vi "Container To String.vi"(0 "variant":variant, 11 "error in (no error)":errorcluster) -> (4 "string":string, 6 "label":string, 15 "error out":errorcluster)   [LabVIEW 2015, in "LV String Utils v1.lvlib"]
doc: "Converts anything to string. String representation is as much compatible with Python repr as possible. Additionally returns label of the wire which is provided at the input."
uses:
  LV String Utils v1.lvlib
  <vilib>/Utility/error.llb/Error Cluster From Error Code.vi
  <vilib>/ErrorRing/Error Ring.xnode
  <vilib>/Utility/Data Type/NI_Data Type.lvlib
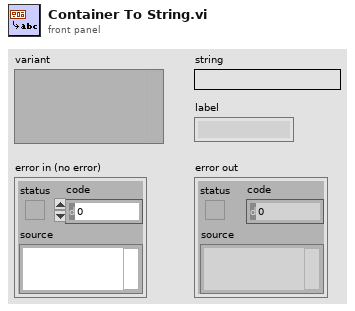
[diagram p1: front panel]
types:
  T1 = typedef "NI_Data Type.lvlib/Data Type.ctl" = enum8{"Invalid Type", "Void", "I8", "I16", "I32", "I64", "U8", "U16", "U32", "U64", "Single Float", "Double Float", "Extended Float", "Single Complex", "Double Complex", "Extended Complex", "Enum U8", "Enum U16", "Enum U32", "Enum U64", "Single Float With Unit", "Double Float With Unit", "Extended Float With Unit", "Single Complex with Unit", "Double Complex with Unit", "Extended Complex with Unit", "Boolean", "String", "Path", "Picture", "Tag", "Array", "Cluster", "Variant", "LV Variant", "Waveform", "Timestamp", "Digital Waveform", "Digital Data", "ExpressData", "Refnum", "External Data", "VI", "Poly VI", "LabVIEW Class Instance", "Fixed Point"}
  T2 = typedef "Refnum Subtype Enum__ogtk.ctl" = enum8{"Generic", "Datalog File Refnum", "Byte Stream File Refnum", "Device Refnum", "Occurence Refnum", "TCP Connection Refnum", "VISA Refnum (Obsolete)", "Automation Renum", "VI Server Refnum", "Menu Refnum", "IVI Refnum (Obsolete)", "IMAQ Session", "0x0C", "Datasocket Refnum", "VISA Resource", "IVI Logical Name", "UDP Connection Refnum", "Notifier Refnum", "Queue Refnum", "IrDA Refnum", "Hardware Plugin Refnum", "Hardware Plugin Tag Refnum", "DAQmx Refnum", "Event Registration Refnum", ".NET Refnum", "User Event Refnum", "0x1A", "Event Callback", "0x1C", "0x1D", "Only Used Internal to LabVIEW", "Bluetooth", "Data Value References", "RT FIFO", "TDM Streaming"}
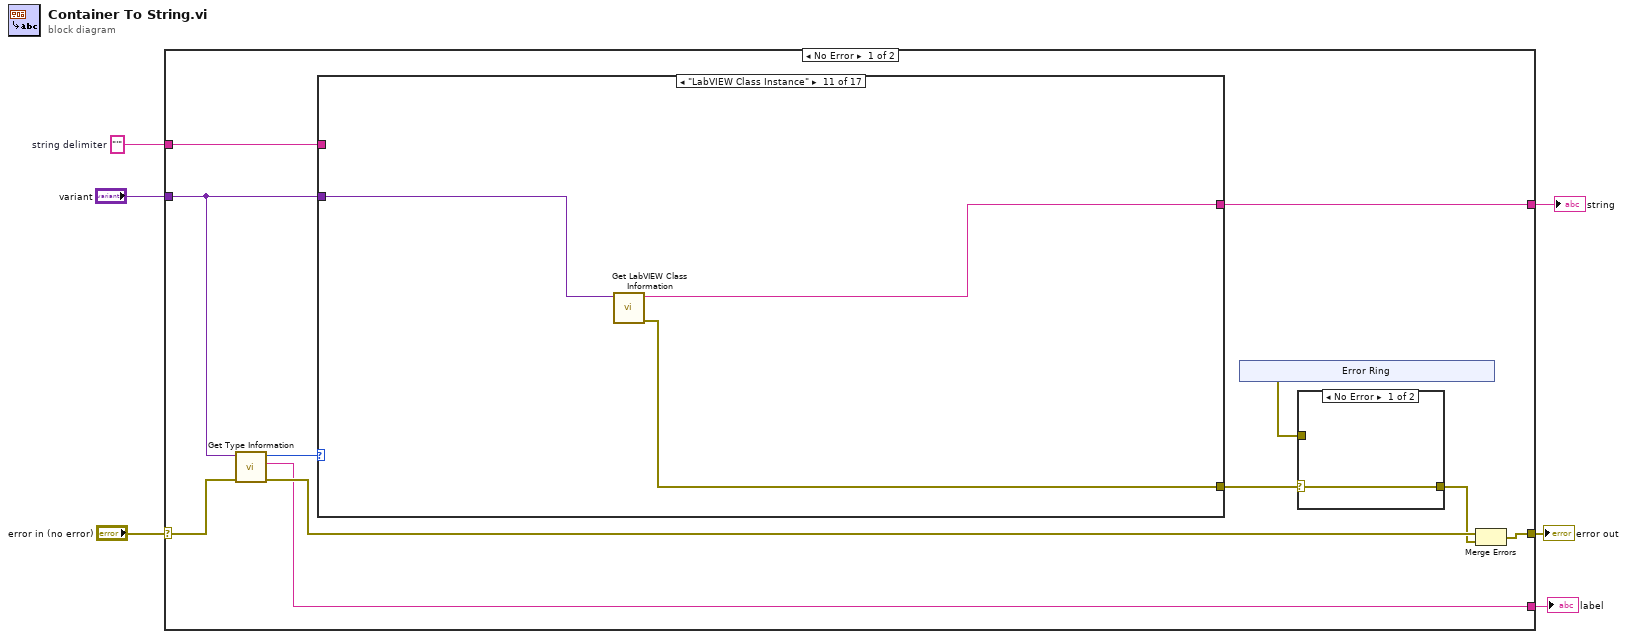
[diagram p0: block diagram]
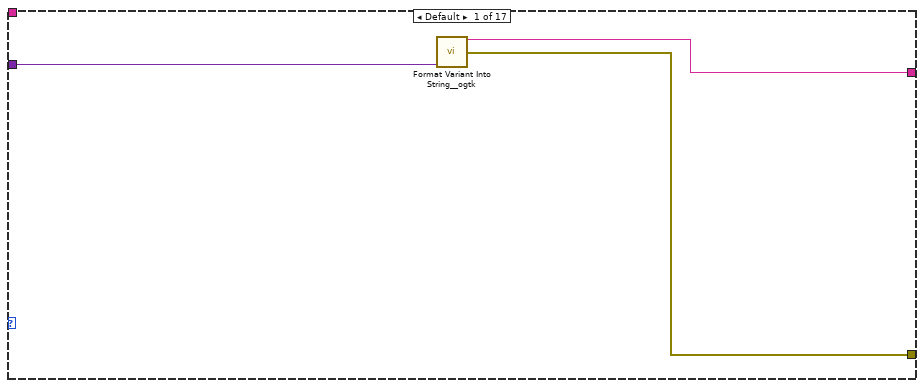
[diagram p3: hidden frame]
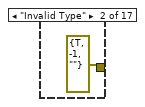
[diagram p4: hidden frame]
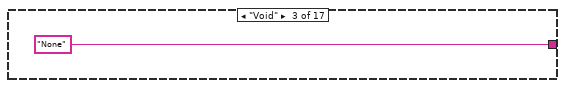
[diagram p5: hidden frame]
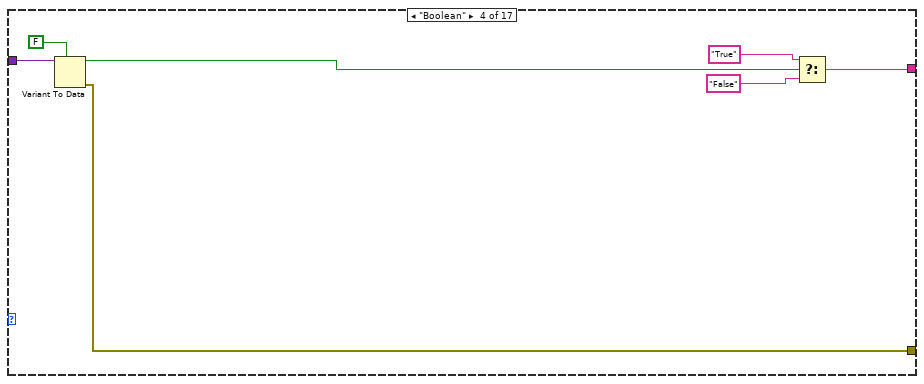
[diagram p6: hidden frame]
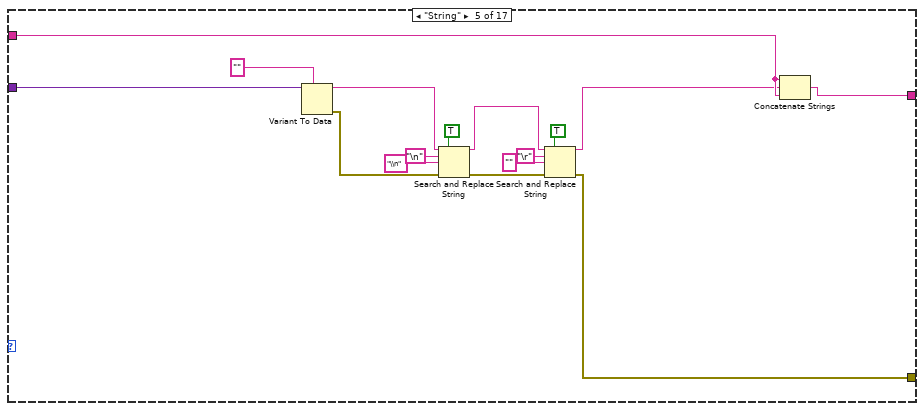
[diagram p7: hidden frame]
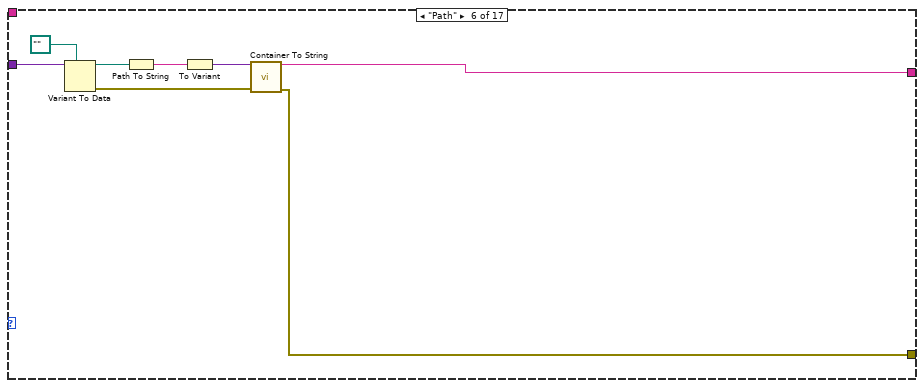
[diagram p8: hidden frame]
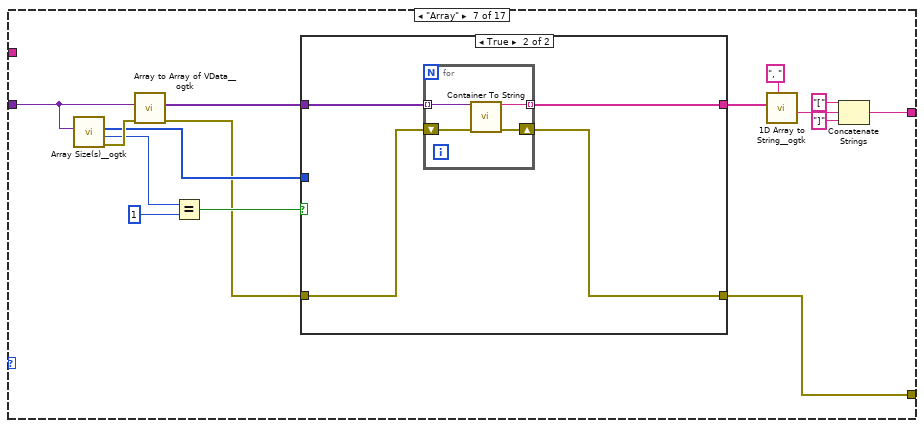
[diagram p9: hidden frame]
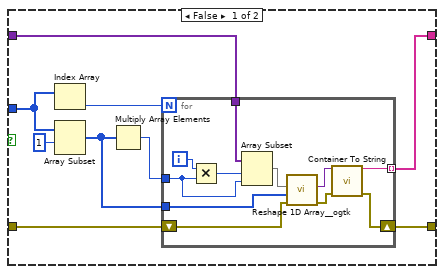
[diagram p10: hidden frame]
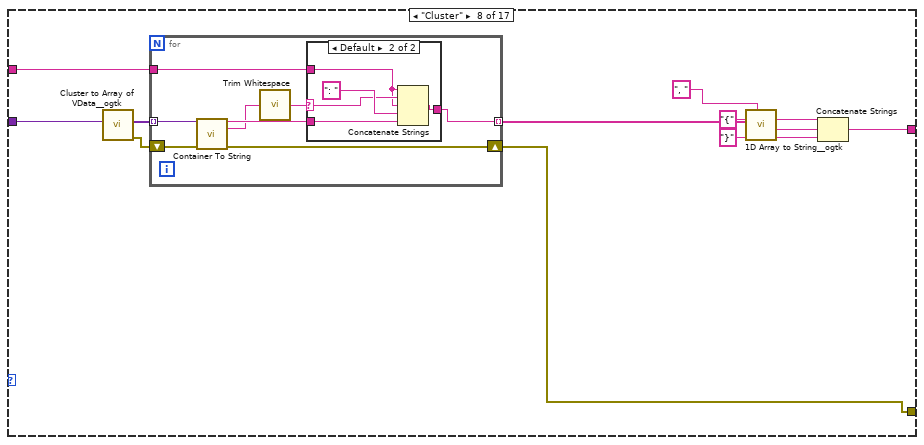
[diagram p11: hidden frame]
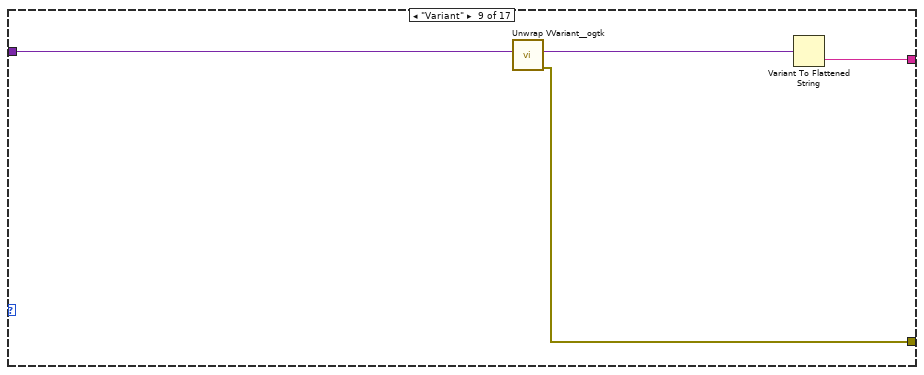
[diagram p13: hidden frame]
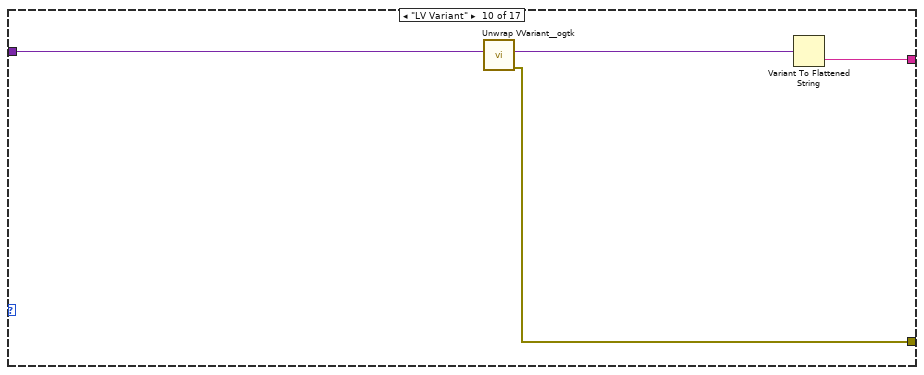
[diagram p14: hidden frame]
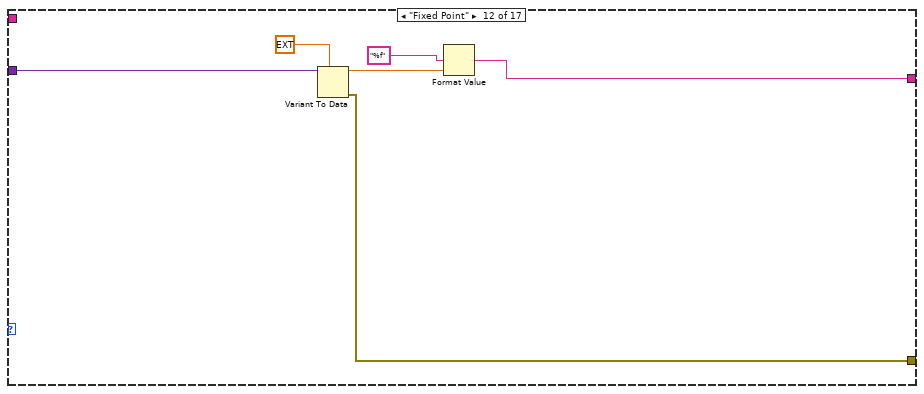
[diagram p15: hidden frame]
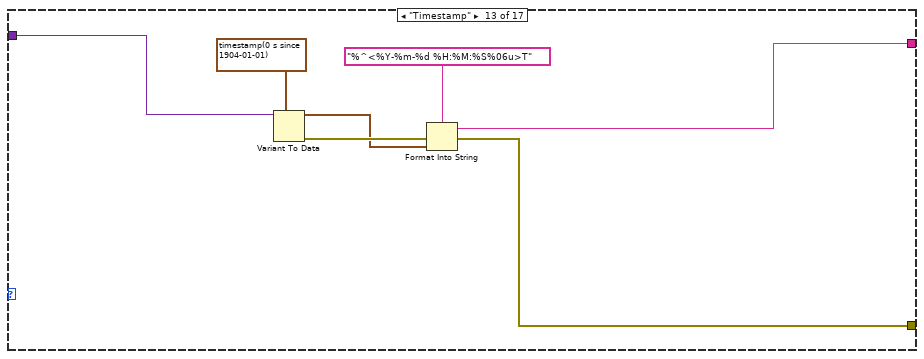
[diagram p16: hidden frame]
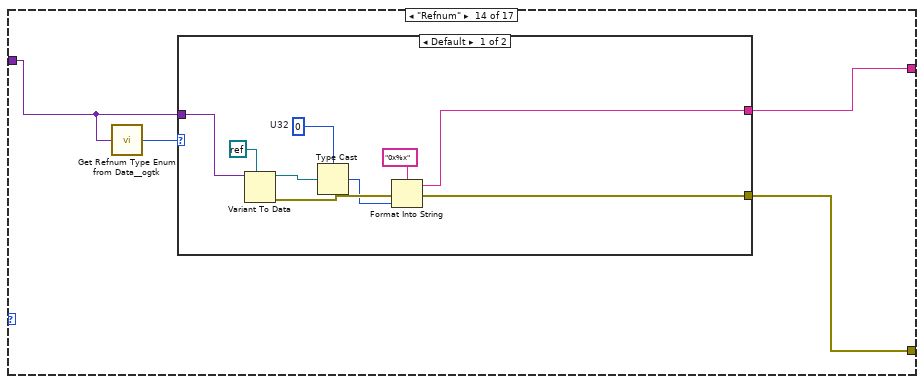
[diagram p17: hidden frame]
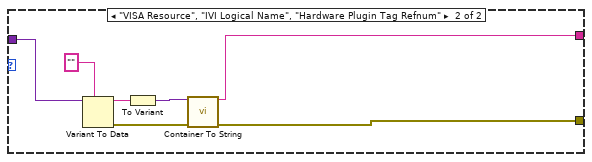
[diagram p18: hidden frame]
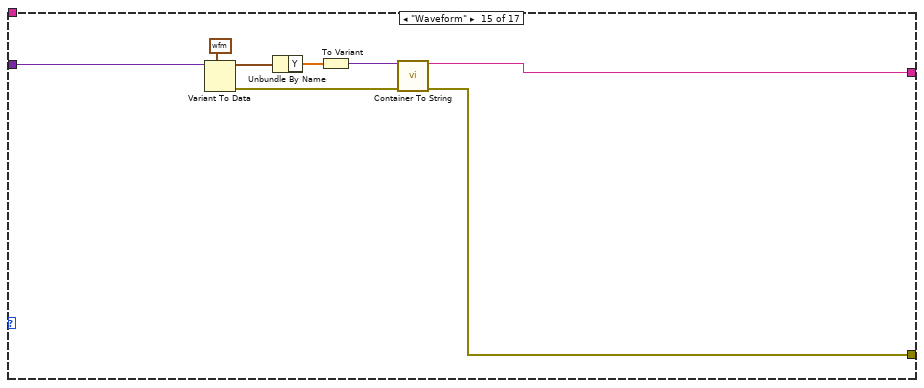
[diagram p19: hidden frame]
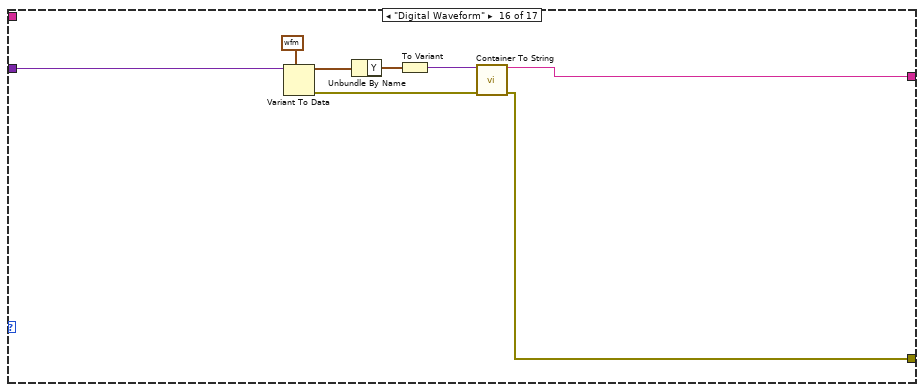
[diagram p20: hidden frame]
diagram:
  w2 = "'"  # string delimiter
  n1 = case shown="No Error" "error in (no error)" {
    selector: "error in (no error)" -> [w10 w196]
    tunnel: [w16 _] -> w6
    tunnel: "variant" -> [w15 _]
    tunnel: [w13 w196] -> w4
    tunnel: [w12 _] -> w3
    tunnel: w2 -> [w11 _]
    frame No Error {
      n2 = call <vilib>:"Get Type Information.vi"("error in (no error)"=w10, "Variant"=w15) -> ("error out"=w14:errorcluster, "Name"=w12:string, "Type"=w17:T1)  [unwired: 5 in, 2 out]
      n3 = case shown="\"LabVIEW Class Instance\"" w17 {
        tunnel: w15 -> [w26 _ _ w34 w51 w58 w66 w108 w130 w134 w137 w144 w150 w155 w179 w183 w194]
        tunnel: [w24 _ "None" ("output string") w32 w49 w54 w65 w104 w131 w135 w136 w140 w145 w153 w172 w180 w188] -> w16
        tunnel: [w25 errorcluster {"status"=TRUE, "code"=-1, "source"=""} ("error out") _ w29 w39 w52 w60 w105 w128 w132 w138 w139 w146 w152 w173 w181 w189] -> w9
        tunnel: w11 -> [_ _ _ _ w48 _ _ w103 _ _ _ _ _ _ _ _ _]
        frame Default {
          n4 = call <userlib>:"Format Variant Into String__ogtk.vi"("Variant"=w26) -> ("Output String"=w24:string, "error out"=w25:errorcluster)  [unwired: 13 in]
        }
        frame "Invalid Type" {
        }
        frame "Void" {
        }
        frame "Boolean" {
          n5 = Variant To Data(type=FALSE, Variant=w34) -> (data=w33:bool, error out=w29:errorcluster)  [unwired: 1 in]
          n6 = Select(t="True", s=w33, f="False") -> (s? t:f=w32:string)
        }
        frame "String" {
          n7 = Variant To Data(type="", Variant=w51) -> (data=w38:string, error out=w40:errorcluster)  [unwired: 1 in]
          n8 = Search and Replace String(replace all?=TRUE ("replace all? (F)"), input string=w38, search string="\n", replace string="\\n" ("replace string (\"\")"), error in=w40) -> (result string=w37:string, error out=w41:errorcluster)  [unwired: 3 in, 2 out]
          n9 = Search and Replace String(replace all?=TRUE ("replace all? (F)"), input string=w37, search string="\r", replace string="" ("replace string (\"\")"), error in=w41) -> (result string=w36:string, error out=w39:errorcluster)  [unwired: 3 in, 2 out]
          n10 = Concatenate Strings(w48, w36, w48) -> (w49:string)
        }
        frame "Path" {
          n11 = Variant To Data(type=path "", Variant=w58) -> (data=w57:path, error out=w53:errorcluster)  [unwired: 1 in]
          n12 = Path To String(path=w57) -> (string=w56:string)
          n13 = To Variant(anything=w56) -> (Variant=w55:variant)
          n14 = call "Container To String.vi"("variant"=w55, "error in (no error)"=w53) -> ("string"=w54:string, "error out"=w52:errorcluster)  [unwired: 11 in, 1 out]
        }
        frame "Array" {
          n15 = call <userlib>:"Array Size(s)__ogtk.vi"("Array"=w66) -> ("error out"=w68:errorcluster, "N dims"=w63:u32, "Size(s)"=w62:u32[])  [unwired: 8 in]
          n16 = call <userlib>:"Array to Array of VData__ogtk.vi"("error in (no error)"=w68, "MultiD Array"=w66) -> ("error out"=w61:errorcluster, "1D Array of Variants"=w69:variant[])  [unwired: 8 in]
          n17 = Equal?(x=w63, y=u32 1) -> (x = y?=w64:bool)
          n18 = case shown="True" w64 {
            tunnel: w69 -> [w83 w98]
            tunnel: w62 -> [w78 _]
            tunnel: [w82 w97] -> w74
            tunnel: w61 -> [w76 w96]
            tunnel: [w75 w95] -> w60
            frame False {
              n19 = Index Array(array=w78) -> (element=w79:u32)  [unwired: 1 in]
              n20 = Array Subset(array=w78, index=1) -> (w77:u32[])  [unwired: 1 in]
              n21 = Multiply Array Elements(1:w77) -> (0:w80:u32)
              n22 = for {
                N: w79 -> [_]
                tunnel: w83 -> [w94]
                tunnel: [w91] -> w82 mode=indexing
                tunnel: w77 -> [w89]
                tunnel: w80 -> [w87]
                shift-right: [w84] -> w75
                shift-left: w76 -> [w85]
                i -> [w93]
                n23 = Multiply(x=w93, y=w87) -> (x*y=w92:u32)
                n24 = Array Subset(array=w94, index=w92, length=w87) -> (w90:variant[])
                n25 = call <userlib>:"Reshape 1D Array__ogtk.vi"("error in (no error)"=w85, "Size(s)"=w89, "1D Array"=w90) -> ("error out"=w86:errorcluster, "Reshaped VArray"=w88:variant)  [unwired: 7 in]
                n26 = call "Container To String.vi"("variant"=w88, "error in (no error)"=w86) -> ("string"=w91:string, "error out"=w84:errorcluster)  [unwired: 11 in, 1 out]
              }
            }
            frame True {
              n27 = for {
                tunnel: w98 -> [w102] mode=indexing
                tunnel: [w101] -> w97 mode=indexing
                shift-right: [w100] -> w95
                shift-left: w96 -> [w99]
                n28 = call "Container To String.vi"("variant"=w102, "error in (no error)"=w99) -> ("string"=w101:string, "error out"=w100:errorcluster)  [unwired: 11 in, 1 out]
              }
            }
          }
          n29 = call <userlib>:"1D Array to String__ogtk.vi"("delimiter (Tab)"=", ", "Array of Strings"=w74) -> ("delimited string"=w72:string)  [unwired: 9 in]
          n30 = Concatenate Strings("[" ("string"), w72, "]" ("string")) -> (w65:string)
        }
        frame "Cluster" {
          n31 = call <userlib>:"Cluster to Array of VData__ogtk.vi"("Cluster"=w108) -> ("error out"=w106:errorcluster, "Array of VData"=w107:variant[])  [unwired: 9 in]
          n32 = for {
            tunnel: w107 -> [w121] mode=indexing
            tunnel: [w117] -> w113 mode=indexing
            shift-right: [w120] -> w105
            shift-left: w106 -> [w119]
            tunnel: w103 -> [w114]
            n33 = call "Container To String.vi"("variant"=w121, "error in (no error)"=w119) -> ("string"=w118:string, "label"=w115:string, "error out"=w120:errorcluster)  [unwired: 11 in]
            n34 = call <vilib>:"Trim Whitespace.vi"("string"=w115) -> ("trimmed string"=w116:string)  [unwired: 1 in]
            n35 = case shown="Default" w116 {
              selector: w116 -> [_ w124]
              tunnel: w118 -> [w122 w127]
              tunnel: [w122 w126] -> w117
              tunnel: w114 -> [_ w123]
              frame "" {
              }
              frame Default {
                n36 = Concatenate Strings(w123, w124, w123, ": " ("string"), w127) -> (w126:string)
              }
            }
          }
          n37 = call <userlib>:"1D Array to String__ogtk.vi"("delimiter (Tab)"=", ", "Array of Strings"=w113) -> ("delimited string"=w111:string)  [unwired: 9 in]
          n38 = Concatenate Strings("{" ("string"), w111, "}" ("string")) -> (w104:string)
        }
        frame "Variant" {
          n39 = call <userlib>:"Unwrap VVariant__ogtk.vi"("VVariant"=w130) -> ("error out"=w128:errorcluster, "Variant"=w129:variant)  [unwired: 9 in]
          n40 = Variant To Flattened String(Variant=w129) -> (data string=w131:string)  [unwired: 1 out]
        }
        frame "LV Variant" {
          n41 = call <userlib>:"Unwrap VVariant__ogtk.vi"("VVariant"=w134) -> ("error out"=w132:errorcluster, "Variant"=w133:variant)  [unwired: 9 in]
          n42 = Variant To Flattened String(Variant=w133) -> (data string=w135:string)  [unwired: 1 out]
        }
        frame "LabVIEW Class Instance" {
          n43 = call <vilib>:"Get LabVIEW Class Information.vi"("Variant"=w137) -> ("error out"=w138:errorcluster, "LabVIEW Class File Name"=w136:string)  [unwired: 8 in, 1 out]
        }
        frame "Fixed Point" {
          n44 = Variant To Data(type=ext 0.0, Variant=w144) -> (data=w141:ext, error out=w139:errorcluster)  [unwired: 1 in]
          n45 = Format Value(format string="%f", value (0)=w141) -> (output string=w140:string)  [unwired: 1 in]
        }
        frame "Timestamp" {
          n46 = Variant To Data(type=timestamp(0 s since 1904-01-01) ("Time Stamp"), Variant=w150) -> (data=w147:timestamp, error out=w148:errorcluster)  [unwired: 1 in]
          n47 = Format Into String(format string="%^<%Y-%m-%d %H:%M:%S%06u>T" ("Format String"), error in=w148, w147) -> (resulting string=w145:string, error out=w146:errorcluster)  [unwired: 1 in]
        }
        frame "Refnum" {
          n48 = call <userlib>:"Get Refnum Type Enum from Data__ogtk.vi"("Data"=w155) -> ("Refnum Subtype Enum"=w154:T2)  [unwired: 4 in]
          n49 = case shown="Default" w154 {
            tunnel: [w157 w168] -> w152
            tunnel: [w158 w167] -> w153
            tunnel: w155 -> [w164 w170]
            frame Default {
              w161 = u32 0  # U32
              n50 = Variant To Data(type=refnum<k0> refnum, Variant=w164) -> (data=w162:refnum<k0>, error out=w160:errorcluster)  [unwired: 1 in]
              n51 = Type Cast(type=w161, x=w162) -> (*(type *) &x=w159:u32)
              n52 = Format Into String(format string="0x%x", error in=w160, w159) -> (resulting string=w158:string, error out=w157:errorcluster)  [unwired: 1 in]
            }
            frame "VISA Resource", "IVI Logical Name", "Hardware Plugin Tag Refnum" {
              n53 = Variant To Data(type="" ("String Value"), Variant=w170) -> (data=w166:string, error out=w169:errorcluster)  [unwired: 1 in]
              n54 = To Variant(anything=w166) -> (Variant=w165:variant)
              n55 = call "Container To String.vi"("variant"=w165, "error in (no error)"=w169) -> ("string"=w167:string, "error out"=w168:errorcluster)  [unwired: 11 in, 1 out]
            }
          }
        }
        frame "Waveform" {
          n56 = Variant To Data(type=waveform(dbl) {"t0"=timestamp(0 s since 1904-01-01), "dt"=1.0, "Y"=[]} ("signal out"), Variant=w179) -> (data=w177:waveform(dbl), error out=w176:errorcluster)  [unwired: 1 in]
          n57 = Unbundle By Name(w177) -> ("Y"=w175:dbl[])
          n58 = To Variant(anything=w175) -> (Variant=w174:variant)
          n59 = call "Container To String.vi"("variant"=w174, "error in (no error)"=w176) -> ("string"=w172:string, "error out"=w173:errorcluster)  [unwired: 11 in, 1 out]
        }
        frame "Digital Waveform" {
          n60 = Variant To Data(type=digitalwaveform {"t0"=timestamp(0 s since 1904-01-01), "dt"=0.0, "Y"={"transitions"=[], "data"=[]}, "error"={"status"=FALSE, "code"=37421928, "source"=""}} ("Digital Waveform"), Variant=w183) -> (data=w187:digitalwaveform, error out=w186:errorcluster)  [unwired: 1 in]
          n61 = Unbundle By Name(w187) -> ("Y"=w185:digitaldata)
          n62 = To Variant(anything=w185) -> (Variant=w184:variant)
          n63 = call "Container To String.vi"("variant"=w184, "error in (no error)"=w186) -> ("string"=w180:string, "error out"=w181:errorcluster)  [unwired: 11 in, 1 out]
        }
        frame "Digital Data" {
          n64 = Variant To Data(type=digitaldata {"transitions"=[], "data"=[]} ("Y"), Variant=w194) -> (data=w192:digitaldata, error out=w195:errorcluster)  [unwired: 1 in]
          n65 = Unbundle By Name(w192) -> ("data"=w191:u8[][])
          n66 = To Variant(anything=w191) -> (Variant=w190:variant)
          n67 = call "Container To String.vi"("variant"=w190, "error in (no error)"=w195) -> ("string"=w188:string, "error out"=w189:errorcluster)  [unwired: 11 in, 1 out]
        }
      }
      n68 = xnode "Error Ring"() -> ("error out"=w7:errorcluster)
      n69 = case shown="No Error" w9 {
        selector: w9 -> [w22 _]
        tunnel: [w22 w23] -> w8
        tunnel: w7 -> [_ w23]
        frame No Error {
        }
        frame Error {
        }
      }
      n70 = Merge Errors(w14, w8) -> (w13:errorcluster)
    }
    frame Error {
    }
  }
  "string" <- w6
  "error out" <- w4
  "label" <- w3
